vi "Subsys02_Global.vi"() -> ()   [LabVIEW 2019]
panel:
  out "S02_V02":dbl
  out "S02_ST":u32(colorbox)
  out "S02_V01":dbl
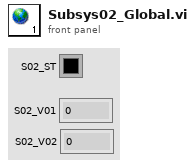
[diagram p1: front panel]
diagram:
